vi "DataVIS_Get_Cursor_Indices.vi"(8 "error in (no error)":errorcluster, 9 "Vslow":dbl[](array[numeric]), 10 "Vfast":dbl[][](array[numeric]), 11 "Cursor Graph":refnum<vi>) -> (0 "error out":errorcluster, 1 "Slow Indices":dbl[](array[numeric]), 2 "Slow Index (Cursor Y)":dbl, 3 "Fast Index (Cursor X) (IDK why it's an array)":dbl[](array[numeric]), 4 "Raw Cursor Position":T1)   [LabVIEW 2016]
uses:
  <vilib>/Utility/miscctls.llb/LVPointDoubleTypeDef.ctl
  <vilib>/gmath/NI_Gmath.lvlib
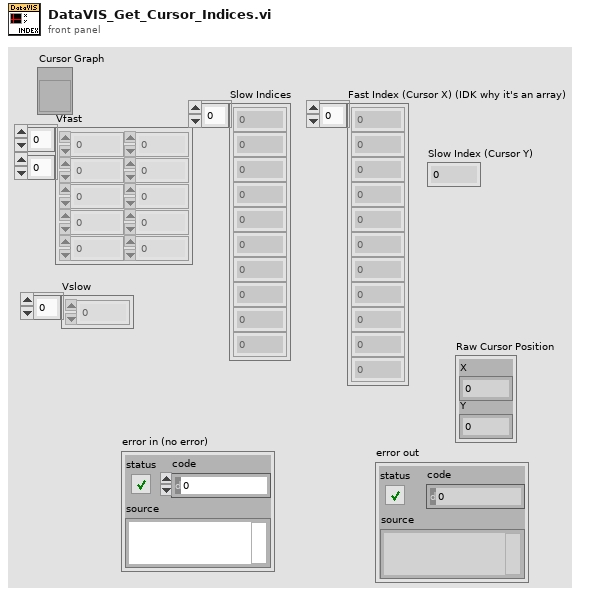
[diagram p1: front panel]
types:
  T1 = typedef "LVPointDoubleTypeDef.ctl" = cluster{"X":dbl, "Y":dbl}
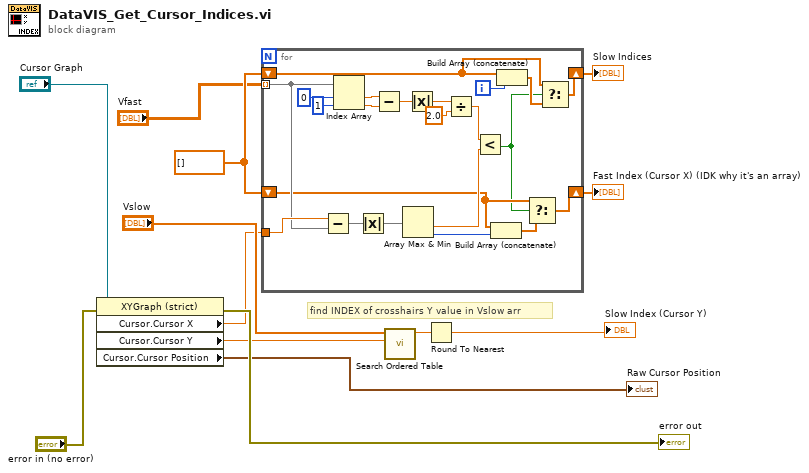
[diagram p0: block diagram]
diagram:
  w13 = dbl[] []
  # "find INDEX of crosshairs Y value in Vslow arr"
  n1 = property class="XYGraph (strict)"(reference="Cursor Graph", error in="error in (no error)") -> (error out=→"error out":errorcluster, "Cursor.Cursor X"=w3:dbl, "Cursor.Cursor Y"=w2:dbl, "Cursor.Cursor Position"=→"Raw Cursor Position":T1)  [unwired: 1 out]
  n2 = for {
    tunnel: "Vfast" -> [w27] mode=indexing
    shift-right: [w14] -> w11
    shift-left: w13 -> [w16]
    shift-right: [w19] -> w10
    shift-left: w13 -> [w20]
    tunnel: w3 -> [w28]
    i -> [w18]
    n3 = Subtract(x=w28, y=w27) -> (x-y=w26:dbl[])
    n4 = Index Array(array=w27, index #1=0 ("index"), index #2=1 ("index")) -> (element #1=w33:dbl, element #2=w32:dbl)
    n5 = Absolute Value(x=w26) -> (abs(x)=w25:dbl[])
    n6 = Subtract(x=w33, y=w32) -> (x-y=w31:dbl)
    n7 = Array Max & Min(array=w25) -> (min value=w23:dbl, min index (indices)=w22:i32)  [unwired: 2 out]
    n8 = Absolute Value(x=w31) -> (abs(x)=w29:dbl)
    n9 = Divide(x=w29, y=2.0) -> (x/y=w24:dbl)
    n10 = Less?(x=w24, y=w23) -> (x < y?=w15:bool)
    n11 = Build Array (concatenate)(w20, w22) -> (w21:dbl[])
    n12 = Build Array (concatenate)(w16, w18) -> (w17:dbl[])
    n13 = Select(t=w20, s=w15, f=w21) -> (s? t:f=w19:dbl[])
    n14 = Select(t=w16, s=w15, f=w17) -> (s? t:f=w14:dbl[])
  }
  "Slow Indices" <- w11
  "Fast Index (Cursor X) (IDK why it's an array)" <- w10
  n15 = call <vilib>:"Search Ordered Table.vi"("x value"=w2, "ordered x array"="Vslow") -> ("fractional index"=w6:dbl)  [unwired: 9 in]
  n16 = Round To Nearest(number=w6) -> (nearest integer value=→"Slow Index (Cursor Y)":dbl)
